vi "Forcade_OffsetPicture.vi"(8 "error in (no error)":errorcluster caption="错误输入（无错误）", 10 "Origin":T1, 11 "Picture_Class 输入":refnum<class "Picture_Class.lvclass"> caption="DNL_LabVIEW Object in") -> (0 "error out":errorcluster caption="错误输出", 3 "Picture_Class 输出":refnum<class "Picture_Class.lvclass"> caption="DNL_LabVIEW Object out")   [LabVIEW 2013, in "Picture_Class.lvclass"]
uses:
  Picture_Class.lvclass
  <vilib>/Utility/miscctls.llb/LVPoint32TypeDef.ctl
  Picture_Class.lvclass/Picture_Class.ctl
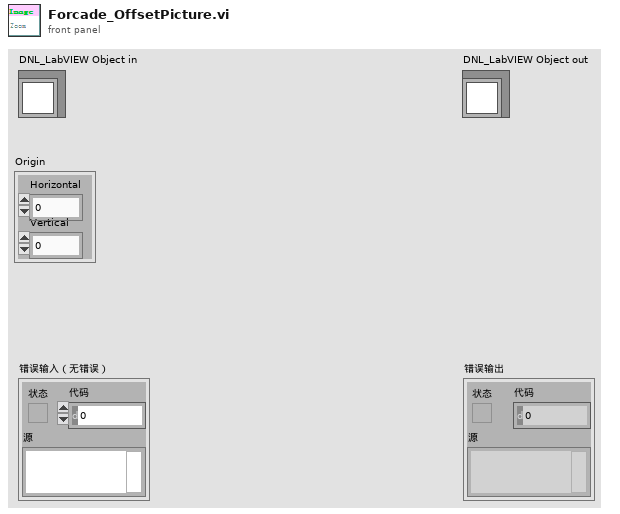
[diagram p1: front panel]
types:
  T1 = typedef "LVPoint32TypeDef.ctl" = cluster{"Horizontal":i32, "Vertical":i32}
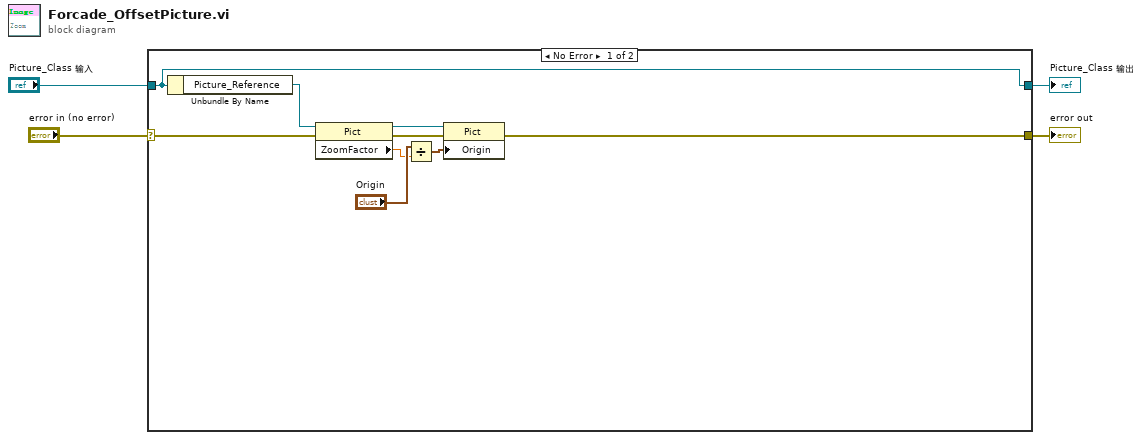
[diagram p0: block diagram]
diagram:
  n1 = case shown="No Error" "error in (no error)" {
    selector: "error in (no error)" -> [w11 w15]
    tunnel: [w8 w15] -> w3
    tunnel: [w13 w14] -> w1
    tunnel: "Picture_Class 输入" -> [w13 w14]
    frame No Error {
      n2 = Unbundle By Name(w13) -> ("Picture_Reference"=w12:refnum<vi>)
      n3 = property class="Pict"(reference=w12, error in=w11) -> (reference out=w10:refnum<vi>, error out=w9:errorcluster, "ZoomFactor"=w5:sgl)
      n4 = Divide(x="Origin", y=w5) -> (x/y=w7:cluster{"Horizontal":sgl, "Vertical":sgl})
      n5 = property class="Pict"(reference=w10, error in=w9, "Origin"=w7) -> (error out=w8:errorcluster)  [unwired: 1 out]
    }
    frame Error {
    }
  }
  "error out" <- w3
  "Picture_Class 输出" <- w1
